vi "TalonSRXReadEncoders.vi"(0 "Device Reference (in)":T1, 1 "Gear Ratio":dbl=1.0, 5 "Simulated Position Goal (deg)":dbl, 7 "Simulated Velocity (deg/s)":dbl=50.0 format="%#_13g", 9 "Simulate":bool, 11 "Error (in)":errorcluster) -> (4 "Device Reference (out)":T1, 6 "Position (deg)":dbl, 8 "Velocity (deg/s)":dbl, 15 "Error (out)":errorcluster)   [LabVIEW 2020]
doc: "Wrapper for reading the integrated encoders from a Talon SRX motor controller. Provides support for simulating the postion of the motor."
uses:
  <vilib>/Rock Robotics/WPI/ThirdParty/Phoenix-LabVIEW/Motor Controller/Get/CTRE_Phoenix_MotorController_GetSelectedSensorData.vi
  <vilib>/Rock Robotics/SystemInterfaces/DIO/FPGA_DIOPWMChannel.ctl
  <vilib>/Rock Robotics/WPI/PWM/WPI_PWMDeadband.ctl
  <vilib>/Rock Robotics/WPI/MotorControl/WPI_MotorControlType.ctl
  <vilib>/Rock Robotics/SystemInterfaces/DIO/FPGA_DIOChannel.ctl
  <vilib>/Rock Robotics/WPI/MotorControl/WPI_MotorControlDeviceRef.ctl
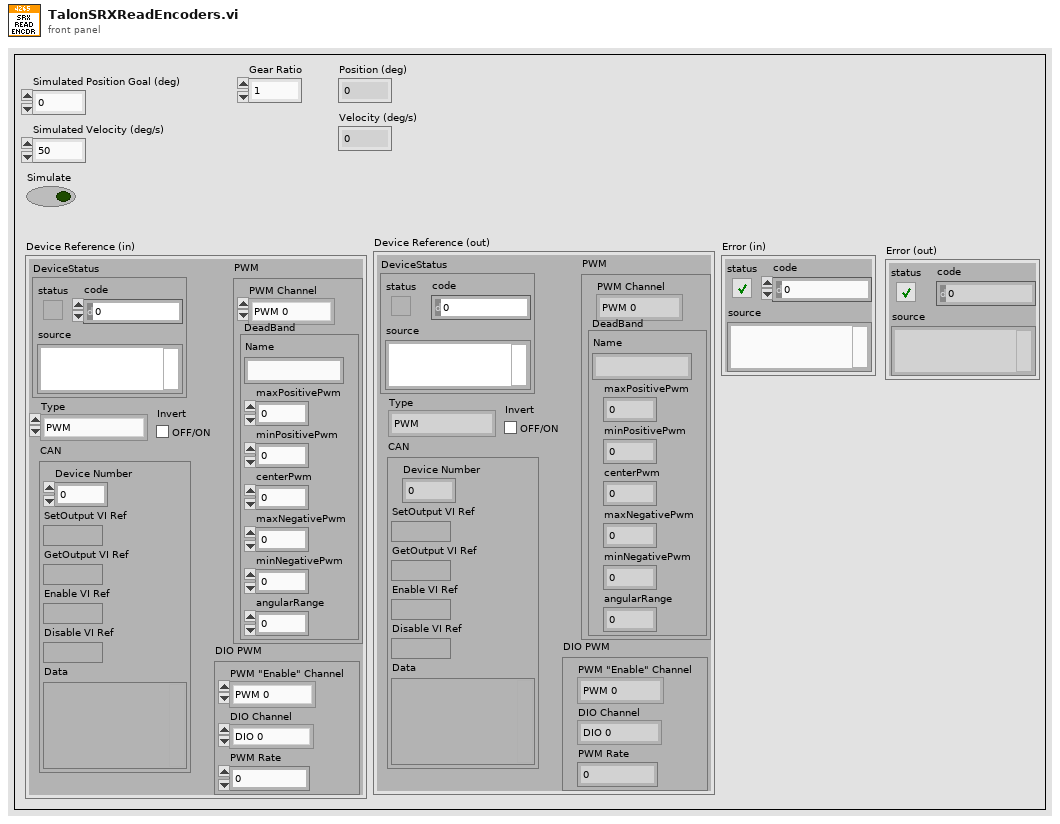
[diagram p1: front panel]
types:
  T1 = typedef "WPI_MotorControlDeviceRef.ctl" = cluster{"DeviceStatus":errorcluster, "Type":T2, "PWM":cluster{"PWM Channel":T3, "DeadBand":T4}, "CAN":cluster{"Device Number":u8, "SetOutput VI Ref":variant, "GetOutput VI Ref":variant, "Enable VI Ref":variant, "Disable VI Ref":variant, "Data":variant}, "Invert":bool, "DIO PWM":cluster{"PWM \"Enable\" Channel":T3, "DIOChannel":T5, "PWM Rate":dbl}}
  T2 = typedef "WPI_MotorControlType.ctl" = enum16{"PWM", "CAN", "DIO PWM"}
  T3 = typedef "FPGA_DIOPWMChannel.ctl" = enum8{"PWM 0", "PWM 1", "PWM 2", "PWM 3", "PWM 4", "PWM 5", "PWM 6", "PWM 7", "PWM 8", "PWM 9", "PWM MXP 0", "PWM MXP 1", "PWM MXP 2", "PWM MXP 3", "PWM MXP 4", "PWM MXP 5", "PWM MXP 6", "PWM MXP 7", "PWM MXP 8", "PWM MXP 9", "Invalid"}
  T4 = typedef "WPI_PWMDeadband.ctl" = cluster{"Name":string, "maxPositivePwm":i32, "minPositivePwm":i32, "centerPwm":i32, "maxNegativePwm":i32, "minNegativePwm":i32, "angularRange":u16}
  T5 = typedef "FPGA_DIOChannel.ctl" = enum8{"DIO 0", "DIO 1", "DIO 2", "DIO 3", "DIO 4", "DIO 5", "DIO 6", "DIO 7", "DIO 8", "DIO 9", "DIO MXP 0", "DIO MXP 1", "DIO MXP 2", "DIO MXP 3", "DIO MXP 4", "DIO MXP 5", "DIO MXP 6", "DIO MXP 7", "DIO MXP 8", "DIO MXP 9", "DIO MXP 10", "DIO MXP 11", "DIO MXP 12", "DIO MXP 13", "DIO MXP 14", "DIO MXP 15", "SPI Port CS1", "SPI Port CS2", "SPI Port CS3", "SPI Port MISO", "SPI Port MOSI", "Invalid"}
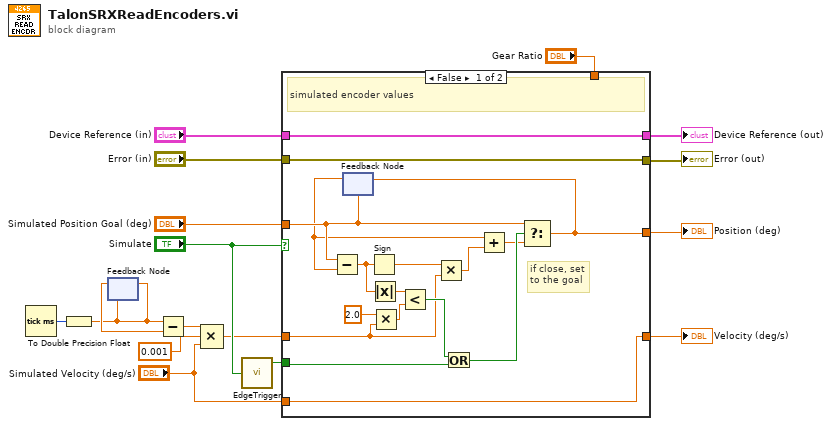
[diagram p0: block diagram]
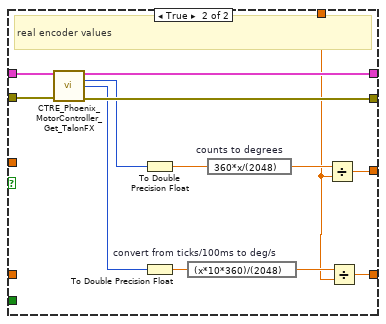
[diagram p2: hidden frame]
diagram:
  n1 = Tick Count (ms)() -> (millisecond timer value=w7:u32)
  n2 = To Double Precision Float(number=w7) -> (double precision float=w5:dbl)
  n3 = feedback-in #1(w5) -> ()
  n4 = feedback #1(w5) -> (w6:dbl)
  n5 = Subtract(x=w5, y=w6) -> (x-y=w4:dbl)
  n6 = Compound Arithmetic op=MULTIPLY(w4, 0.001 ("value"), "Simulated Velocity (deg/s)") -> (w2:dbl)
  n7 = call "EdgeTrigger.vi"("Input Signal"="Simulate") -> ("Rising Edge Trigger"=w14:bool)  [unwired: 2 out]
  n8 = case shown="False" "Simulate" {
    tunnel: [w22 w47] -> w11
    tunnel: [w21 w46] -> w12
    tunnel: [w20 w40] -> w9
    tunnel: [w18 w36] -> w8
    tunnel: "Device Reference (in)" -> [w22 w45]
    tunnel: "Error (in)" -> [w21 w44]
    tunnel: w14 -> [w34 _]
    tunnel: "Simulated Position Goal (deg)" -> [w33 _]
    tunnel: "Gear Ratio" -> [_ w35]
    tunnel: w2 -> [w19 _]
    tunnel: "Simulated Velocity (deg/s)" -> [w18 _]
    frame False {
      # "if close, set\nto the goal"
      # "simulated encoder values"
      n9 = feedback #2(w33) -> (w28:dbl)
      n10 = Subtract(x=w33, y=w28) -> (x-y=w27:dbl)
      n11 = Sign(1:w27) -> (0:w30:dbl)
      n12 = Absolute Value(x=w27) -> (abs(x)=w26:dbl)
      n13 = Multiply(x=2.0, y=w19) -> (x*y=w25:dbl)
      n14 = Less?(x=w26, y=w25) -> (x < y?=w32:bool)
      n15 = Multiply(x=w30, y=w19) -> (x*y=w29:dbl)
      n16 = Or(x=w32, y=w34) -> (x .or. y?=w31:bool)
      n17 = Add(x=w28, y=w29) -> (x+y=w23:dbl)
      n18 = Select(t=w33, s=w31, f=w23) -> (s? t:f=w20:dbl)
      n19 = feedback-in #2(w20) -> ()
    }
    frame True {
      # "real encoder values"
      n20 = call-poly <vilib>:"CTRE_Phoenix_MotorController_Get_TalonFX.vi"("PhoenixMotorControlDevRef"=w45, "error in"=w44) -> ("PhoenixMotorControlDevRef"=w47:T1, "Position (Raw Sensor Units)"=w41:i32, "Velocity (Raw Sensor Units per 100 ms)"=w37:i32, "error out"=w46:errorcluster)  [unwired: 10 in]
      n21 = To Double Precision Float(number=w41) -> (double precision float=w42:dbl)
      n22 = To Double Precision Float(number=w37) -> (double precision float=w39:dbl)
      n23 = expression code="(x*10*360)/(2048)" "convert from ticks/100ms to deg/s"(w39) -> (w38:dbl)
      n24 = expression code="360*x/(2048)" "counts to degrees"(w42) -> (w43:dbl)
      n25 = Divide(x=w43, y=w35) -> (x/y=w40:dbl)
      n26 = Divide(x=w38, y=w35) -> (x/y=w36:dbl)
    }
  }
  "Position (deg)" <- w9
  "Velocity (deg/s)" <- w8
  "Error (out)" <- w12
  "Device Reference (out)" <- w11
